vi "Read On Board Memory (NVM).vi"(0 "Session Handle in":T1, 1 "Reverse?":bool, 5 "Address":u16=171 format="%x", 11 "error in (no error)":errorcluster) -> (4 "Session Handle out":T1, 6 "Read Bytes":u8[](array[numeric]), 15 "error out":errorcluster)   [LabVIEW 2015, in "PAS.lvclass"]
uses:
  PAS.lvclass
  Typedefs/Session Handle.ctl
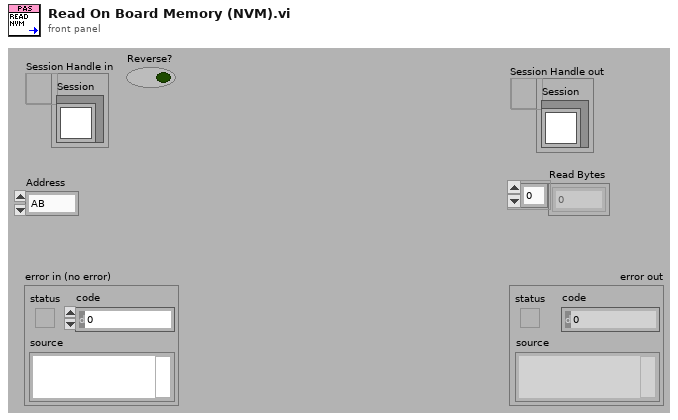
[diagram p1: front panel]
types:
  T1 = typedef "PAS.lvclass/Session Handle.ctl" = refnum<data-value>
  T2 = typedef "XNET Frame CAN.ctl" = cluster{"timestamp":timestamp, "payload":u8[], "identifier":u32, "type":T3, "extended?":bool, "echo?":bool}
  T3 = typedef "XNET Frame Type CAN.ctl" = u8
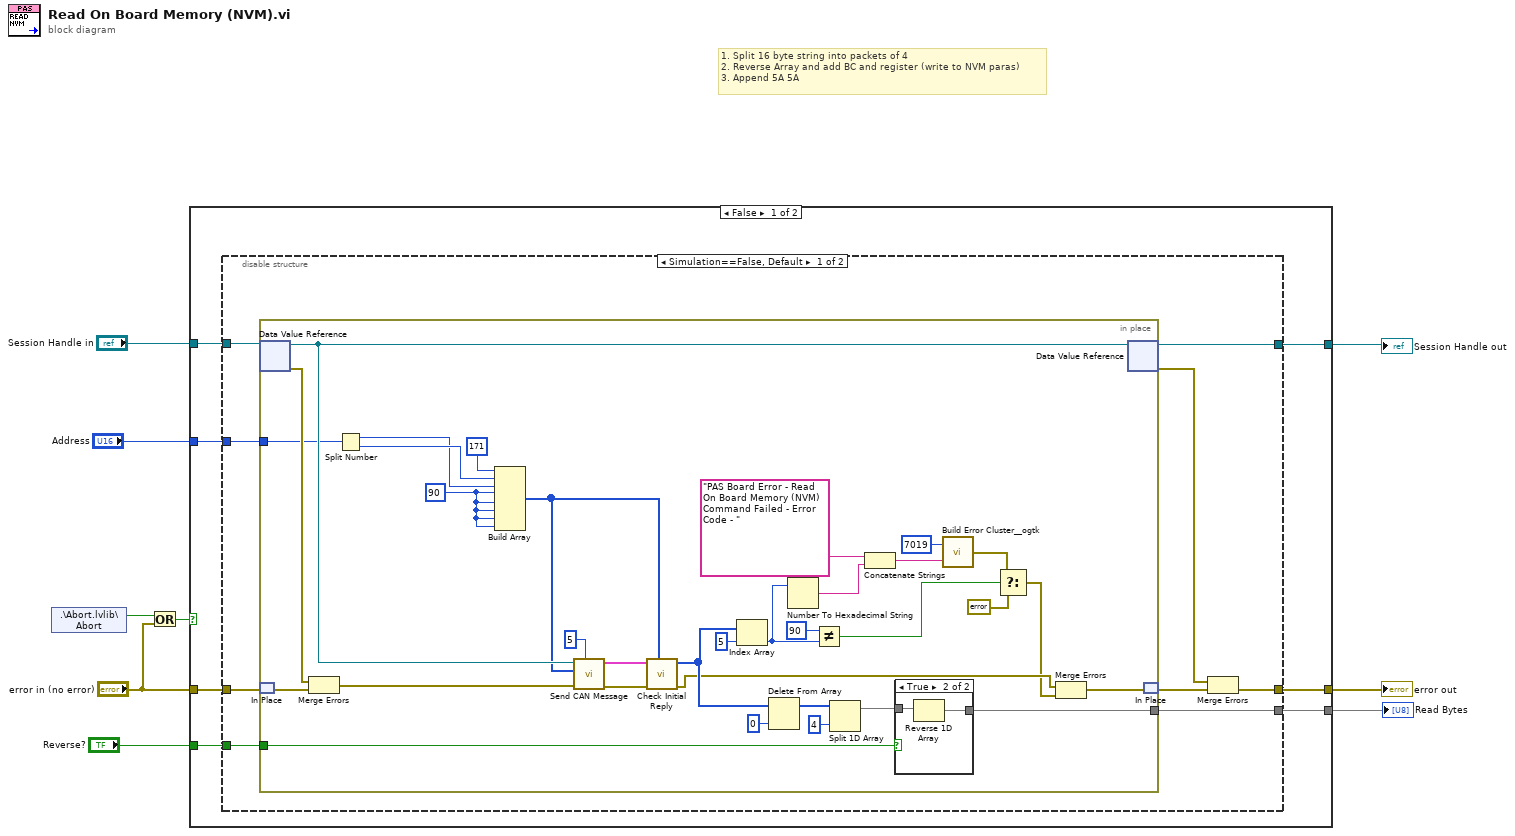
[diagram p0: block diagram]
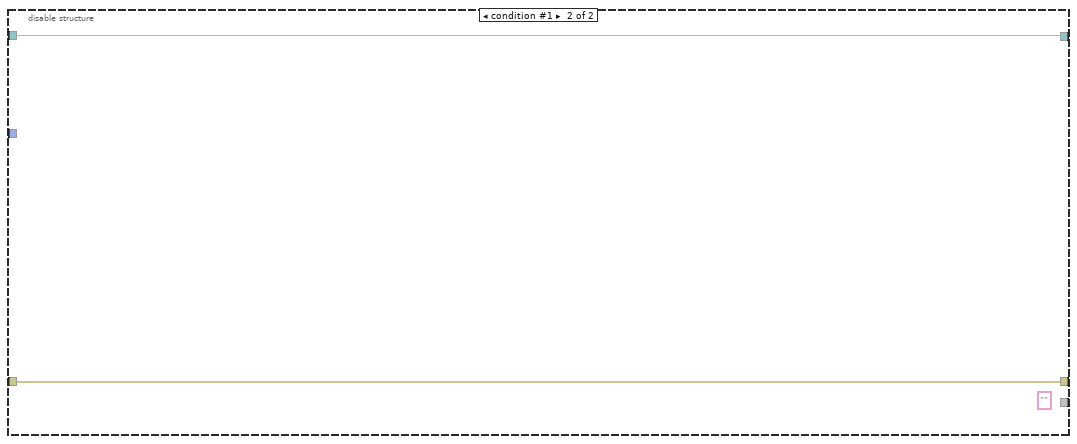
[diagram p3: hidden frame]
diagram:
  # "1. Split 16 byte string into packets of 4\n2. Reverse Array and add BC and register (write to NVM paras)\n3. Append 5A 5A"
  n1 = shared-variable ".\\Abort.lvlib\\Abort"() -> (w6:bool)  [unwired: 1 in, 1 out]
  n2 = Or(x=w6, y="error in (no error)") -> (x .or. y?=w4:bool)
  n3 = case shown="False" w4 {
    tunnel: [w16 w65] -> w8
    tunnel: [w15 w64] -> w7
    tunnel: "Session Handle in" -> [w14 w65]
    tunnel: "error in (no error)" -> [w13 w64]
    tunnel: "Address" -> [w12 _]
    tunnel: [w11 _] -> w2
    tunnel: "Reverse?" -> [w10 _]
    frame False {
      n4 = disable-structure shown="Simulation==False, Default" {
        disable-tunnel: [w25 w63] -> w16
        disable-tunnel: [w22 w62] -> w15
        disable-tunnel: w14 -> [w21 w63]
        disable-tunnel: w13 -> [w20 w62]
        disable-tunnel: w12 -> [w19 _]
        disable-tunnel: [w18 _] -> w11
        disable-tunnel: w10 -> [w17 _]
        frame condition #0 (active) {
          n5 = in-place {
            in-place-border: w19 -> [w44]
            in-place-border: [w40] -> w18
            in-place-border: w17 -> [w26]
            w41 = u8 90
            n6 = in-place-dvr #1(w21) -> (w55:refnum<class "PAS.lvclass">, w58:errorcluster)
            n7 = in-place-match #2(w20) -> (w57:errorcluster)
            n8 = Merge Errors(w58, w57) -> (w56:errorcluster)
            n9 = Split Number(x=w44) -> (hi(x)=w42:u8, lo(x)=w43:u8)
            n10 = Build Array(u8 171, w43, w42, w41, w41, w41, w41, w41) -> (w50:u8[])
            n11 = call "Send CAN Message.vi"("Number of Retries"=5, "error in (no error)"=w56, "payload"=w50, "Gas In"=w55) -> ("error out"=w29:errorcluster, "Reply"=w51:T2[])  [unwired: 5 in, 1 out]
            n12 = call "Check Initial Reply.vi"("Write Message"=w50, "error in (no error)"=w29, "Reply"=w51) -> ("error out"=w28:errorcluster, "Data Packet"=w30:u8[])  [unwired: 5 in, 2 out]
            n13 = Index Array(array=w30, index=5) -> (element=w36:u8)
            n14 = Delete From Array(array=w30, index=0) -> (array with subset deleted=w31:u8[])  [unwired: 1 in, 1 out]
            n15 = Number To Hexadecimal String(2:w36) -> (0:w35:string)  [unwired: 1 in]
            n16 = Not Equal?(x=u8 90, y=w36) -> (x != y?=w33:bool)
            n17 = Split 1D Array(array=w31, index=4) -> (first subarray=w45:u8[])  [unwired: 1 out]
            n18 = Concatenate Strings("PAS Board Error - Read On Board Memory (NVM) Command Failed - Error Code - " ("string"), w35) -> (w34:string)
            n19 = case shown="True" w26 {
              tunnel: w45 -> [w59 w61]
              tunnel: [w59 w60] -> w40
              frame False {
              }
              frame True {
                n20 = Reverse 1D Array(array=w61) -> (reversed array=w60:u8[])
              }
            }
            n21 = call <userlib>:"Build Error Cluster__ogtk.vi"("String to Prepend to source (\"\")"=w34, "code"=7019) -> ("error out"=w48:errorcluster)
            n22 = Select(t=w48, s=w33, f=errorcluster {"status"=FALSE, "code"=0, "source"=""}) -> (s? t:f=w27:errorcluster)
            n23 = Merge Errors(w28, w27) -> (w54:errorcluster)
            n24 = in-place-dvr #1(w55) -> (w25:T1, w23:errorcluster)
            n25 = in-place-match #2(w54) -> (w24:errorcluster)
          }
          n26 = Merge Errors(w23, w24) -> (w22:errorcluster)
        }
        frame condition #1 {
          (unwired) "" ("string")
        }
      }
    }
    frame True {
    }
  }
  "Session Handle out" <- w8
  "error out" <- w7
  "Read Bytes" <- w2
